vi "runCTempController.vi"(8 "error in (no error)":errorcluster) -> (0 "error out":errorcluster)   [LabVIEW 2009, in "iManagement.lvlib" / "CameraManager.lvclass"]
uses:
  CameraManager.lvclass
  CameraManager.lvclass/CameraManager.ctl
  Hal/Channels/Camera/CameraController.lvclass
  Hal/Channels/Camera/CameraEventsManager/CameraEventsManger.lvclass
  Hal/Channels/Camera/CameraTempControllerRunner.lvclass
panel:
  in  "CameraManager.lvclass":refnum<class "CameraManager.lvclass">
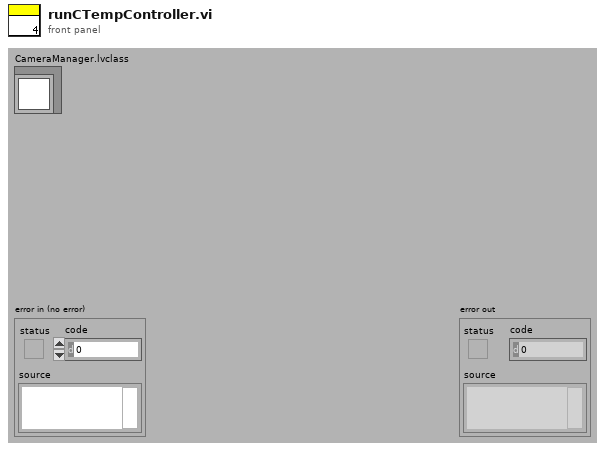
[diagram p1: front panel]
types:
  T1 = cluster{"newSetPointEvent":refnum<user-event>, "stopCoolingEvent":refnum<user-event>}
  T2 = cluster{"closeEvent":refnum<user-event>, "temperatureUpdateEvent":refnum<user-event>, "displayErrorEvent":refnum<user-event>, "setPointUpdateEvent":refnum<user-event>}
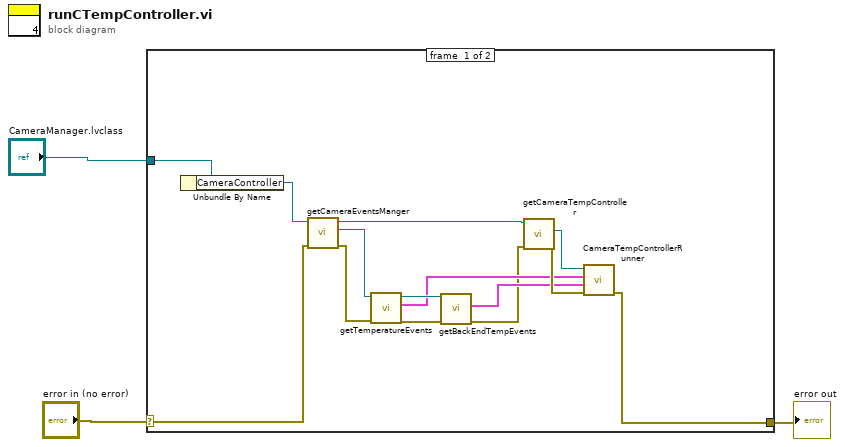
[diagram p0: block diagram]
diagram:
  n1 = case shown="No Error" "error in (no error)" {
    selector: "error in (no error)" -> [w17 w18]
    tunnel: [w4 w18] -> w2
    tunnel: "CameraManager.lvclass" -> [w13 _]
    frame #0 {
      n2 = Unbundle By Name(w13) -> ("CameraController"=w12:refnum<class "CameraController.lvclass">)
      n3 = call-dynamic "getCameraEventsManger.vi"("error in (no error)"=w17, "CameraController.lvclass in"=w12) -> ("error out"=w6:errorcluster, "Hardware:Channels.lvlib:CameraEventsManger.lvclass"=w11:refnum<class "CameraEventsManger.lvclass">, "CameraController.lvclass out"=w16:refnum<class "CameraController.lvclass">)  [unwired: 7 in]
      n4 = call-dynamic "getTemperatureEvents.vi"("error in (no error)"=w6, "CameraEventsManger.lvclass in"=w11) -> ("error out"=w7:errorcluster, "temperatureEvents"=w9:T1, "CameraEventsManger.lvclass out"=w10:refnum<class "CameraEventsManger.lvclass">)  [unwired: 7 in]
      n5 = call-dynamic "getBackEndTempEvents.vi"("error in (no error)"=w7, "CameraEventsManger.lvclass in"=w10) -> ("error out"=w5:errorcluster, "backEndTempEvents"=w8:T2)  [unwired: 7 in, 1 out]
      n6 = call-dynamic "getCameraTempController.vi"("error in (no error)"=w5, "CameraController.lvclass in"=w16) -> ("error out"=w14:errorcluster, "Hardware:Channels.lvlib:CameraTempController.lvclass"=w15:refnum<class "CameraTempController.lvclass">)  [unwired: 7 in, 1 out]
      n7 = call "CameraTempControllerRunner.vi"("error in (no error)"=w14, "tempControllerBackEndEvents in"=w8, "tempControllerFrontEndEvents in"=w9, "CameraTempController"=w15) -> ("error out"=w4:errorcluster)  [unwired: 4 in, 3 out]
    }
    frame #1 {
    }
  }
  "error out" <- w2
